vi "save_infos_svi.vi"(0 "Refnum VISA en entrée":refnum<visa-resource-name>="COM1", 1 "SOFT_VERSION":string="V2", 2 "Noff":u32 step=1, 3 "Camera Model":string="f", 4 "Non":u32=150 step=1, 5 "Camera Serial":string="f", 6 "Nstart":u32=30 step=1, 8 "USED_FILTERS":u8[](array[numeric]), 9 "Version":string="f", 10 "info Directory":path=path "D:/CONFIGS_TIME_LAPSE", 11 "STAGE_SPEED":dbl, 12 "ROMODE":u32, 13 "NSCAN":u32, 14 "BIN":u16, 15 "BETWEEN_SCAN":u32, 16 "EXPT":dbl, 17 "NPAT":u32, 18 "USED_LEDS":bool[][](array[boolean])=[[FALSE, FALSE], [TRUE, TRUE]], 19 "BETWEEN_PAT":u32) -> ()   [LabVIEW 2013]
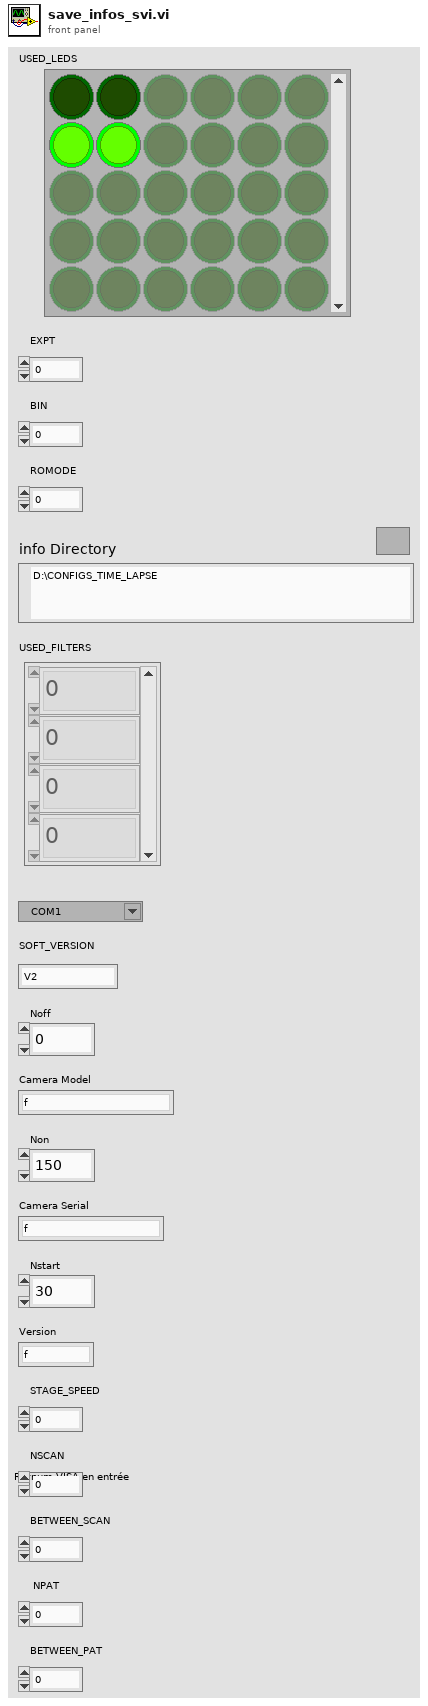
[diagram p1: front panel]
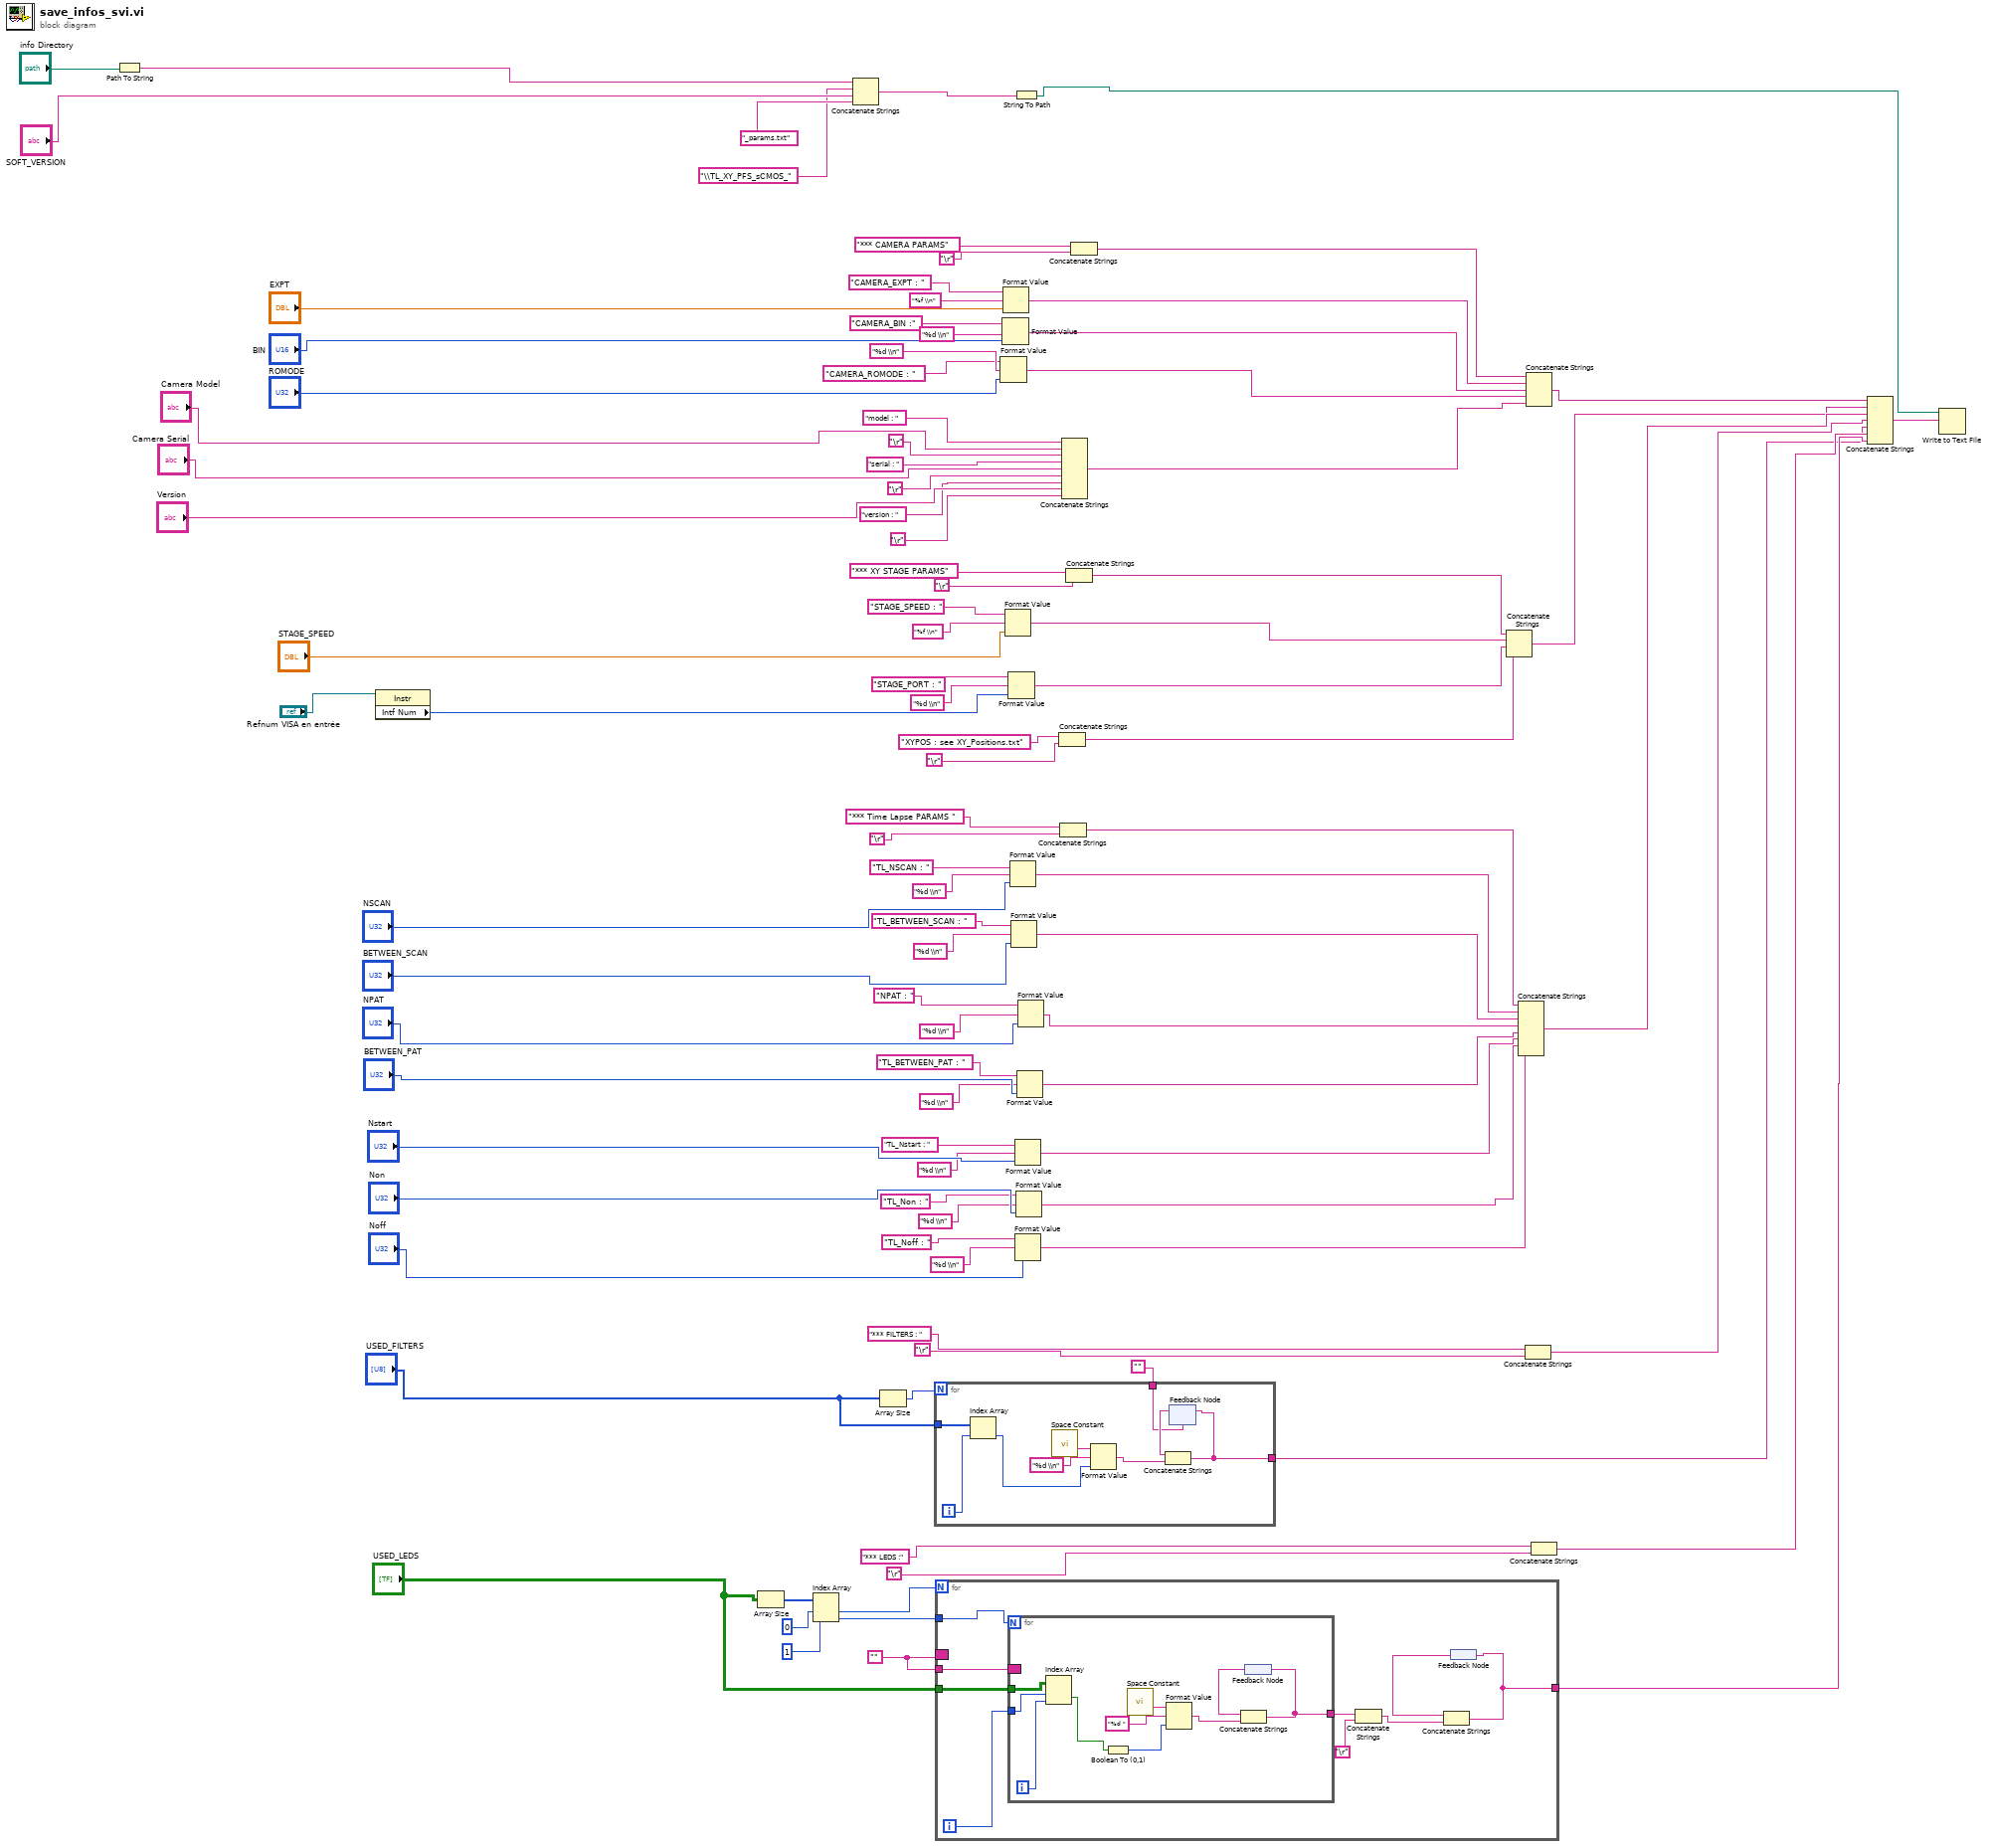
[diagram p0: block diagram]
diagram:
  w100 = ""
  n1 = Path To String(path="info Directory") -> (string=w2:string)
  n2 = property class="Instr"(reference="Refnum VISA en entrée") -> ("Intf Num"=w27:u16)  [unwired: 1 in, 2 out]
  n3 = Array Size(array="USED_LEDS") -> (size(s)=w66:i32[])
  n4 = Index Array(array=w66, index #1=0, index #2=1) -> (element #1=w67:i32, element #2=w99:i32)
  n5 = Concatenate Strings(w2, "\\TL_XY_PFS_sCMOS_", "SOFT_VERSION", "_params.txt") -> (w6:string)
  n6 = Array Size(array="USED_FILTERS") -> (size(s)=w61:i32)
  n7 = for {
    N: w61 -> [_]
    tunnel: "USED_FILTERS" -> [w106]
    tunnel: "" -> [w102]
    tunnel: [w101] -> w90
    i -> [w107]
    n8 = Index Array(array=w106, index=w107) -> (element=w105:u8)
    n9 = call <vilib>:"Space Constant.vi"() -> ("String"=w108:string)
    n10 = Format Value(string ("")=w108, format string="%d \\n", value (0)=w105) -> (output string=w104:string)
    n11 = feedback #1(w102) -> (w103:string)
    n12 = Concatenate Strings(w103, w104) -> (w101:string)
    n13 = feedback-in #1(w101) -> ()
  }
  n14 = for {
    N: w67 -> [_]
    tunnel: "USED_LEDS" -> [w118]
    tunnel: [w112] -> w92
    tunnel: w99 -> [w111]
    border: w100 -> [_]
    tunnel: w100 -> [w110]
    i -> [w117]
    n15 = for {
      N: w111 -> [_]
      tunnel: w118 -> [w127]
      tunnel: w117 -> [w119]
      tunnel: [w121] -> w115
      border: w110 -> [_]
      i -> [w120]
      n16 = Index Array(array=w127, index (row)=w119, index (col)=w120) -> (element=w125:bool)
      n17 = Boolean To (0,1)(Boolean=w125) -> (0, 1=w124:i16)
      n18 = call <vilib>:"Space Constant.vi"() -> ("String"=w126:string)
      n19 = Format Value(string ("")=w126, format string="%d ", value (0)=w124) -> (output string=w123:string)
      n20 = feedback #2() -> (w122:string)
      n21 = Concatenate Strings(w122, w123) -> (w121:string)
      n22 = feedback-in #2(w121) -> ()
    }
    n23 = Concatenate Strings(w115, "\r") -> (w114:string)
    n24 = feedback #3() -> (w113:string)
    n25 = Concatenate Strings(w113, w114) -> (w112:string)
    n26 = feedback-in #3(w112) -> ()
  }
  n27 = Format Value(string ("")="CAMERA_ROMODE : ", format string="%d \\n", value (0)="ROMODE") -> (output string=w84:string)
  n28 = Format Value(string ("")="CAMERA_BIN :", format string="%d \\n", value (0)="BIN") -> (output string=w83:string)
  n29 = Format Value(string ("")="CAMERA_EXPT : ", format string="%f \\n", value (0)="EXPT") -> (output string=w82:string)
  n30 = Format Value(string ("")="STAGE_SPEED : ", format string="%f \\n", value (0)="STAGE_SPEED") -> (output string=w79:string)
  n31 = Format Value(string ("")="STAGE_PORT : ", format string="%d \\n", value (0)=w27) -> (output string=w80:string)
  n32 = Format Value(string ("")="TL_NSCAN : ", format string="%d \\n", value (0)="NSCAN") -> (output string=w71:string)
  n33 = Format Value(string ("")="TL_BETWEEN_SCAN : ", format string="%d \\n", value (0)="BETWEEN_SCAN") -> (output string=w72:string)
  n34 = String To Path(string=w6) -> (path=w94:path)
  n35 = Format Value(string ("")="TL_Nstart : ", format string="%d \\n", value (0)="Nstart") -> (output string=w75:string)
  n36 = Format Value(string ("")="TL_Noff : ", format string="%d \\n", value (0)="Noff") -> (output string=w77:string)
  n37 = Format Value(string ("")="TL_Non : ", format string="%d \\n", value (0)="Non") -> (output string=w76:string)
  n38 = Format Value(string ("")="TL_BETWEEN_PAT : ", format string="%d \\n", value (0)="BETWEEN_PAT") -> (output string=w74:string)
  n39 = Format Value(string ("")="NPAT : ", format string="%d \\n", value (0)="NPAT") -> (output string=w73:string)
  n40 = Concatenate Strings("XYPOS : see XY_Positions.txt", "\r") -> (w97:string)
  n41 = Concatenate Strings("*** Time Lapse PARAMS ", "\r") -> (w70:string)
  n42 = Concatenate Strings("model : ", "Camera Model", "\r", "serial : ", "Camera Serial", "\r", "version : ", "Version", "\r") -> (w85:string)
  n43 = Concatenate Strings("*** XY STAGE PARAMS", "\r") -> (w78:string)
  n44 = Concatenate Strings("*** CAMERA PARAMS", "\r") -> (w81:string)
  n45 = Concatenate Strings(w78, w79, w80, w97) -> (w87:string)
  n46 = Concatenate Strings(w70, w71, w72, w73, w74, w75, w76, w77) -> (w88:string)
  n47 = Concatenate Strings("*** FILTERS : ", "\r") -> (w89:string)
  n48 = Concatenate Strings(w81, w82, w83, w84, w85) -> (w86:string)
  n49 = Concatenate Strings("*** LEDS :", "\r") -> (w91:string)
  n50 = Concatenate Strings(w86, w87, w88, w89, w90, w91, w92) -> (w93:string)
  n51 = Write to Text File(file (use dialog)=w94, text=w93) -> ()  [unwired: 2 in, 3 out]
